vi "Select Pixel from MUX.vi"(7 "Cell position":dbl, 9 "Pixel":i32, 10 "Sample Holder":dbl) -> ()   [LabVIEW 2011]
uses:
  <vilib>/ULx/Create Channel.llb/ULx Create Channel (DO-Digital Output).vi
  <vilib>/ULx/Write.llb/ULx Write (Digital U32 1Chan 1Samp).vi
panel:
  in  "Port":refnum<k21>="Dev0/AuxPort"
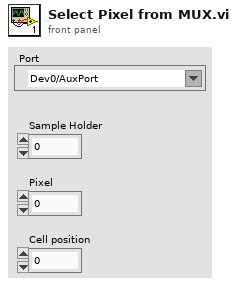
[diagram p1: front panel]
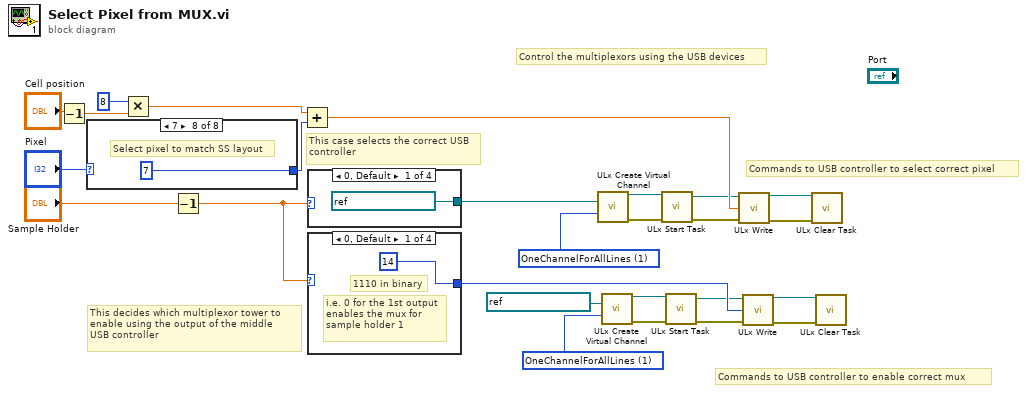
[diagram p0: block diagram]
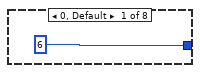
[diagram p2: hidden frame]
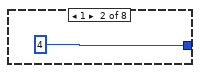
[diagram p3: hidden frame]
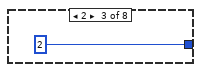
[diagram p4: hidden frame]
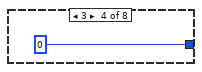
[diagram p5: hidden frame]
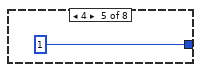
[diagram p6: hidden frame]
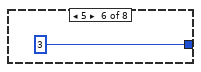
[diagram p7: hidden frame]
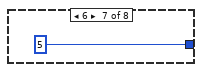
[diagram p8: hidden frame]
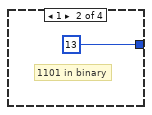
[diagram p9: hidden frame]
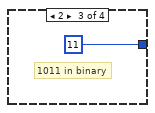
[diagram p10: hidden frame]
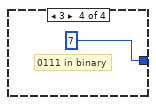
[diagram p11: hidden frame]
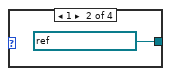
[diagram p12: hidden frame]
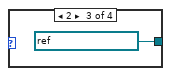
[diagram p13: hidden frame]
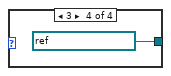
[diagram p14: hidden frame]
diagram:
  w15 = 1 items=["OneChannelForEachLine", "OneChannelForAllLines"] ("line grouping")
  w2 = 1 items=["OneChannelForEachLine", "OneChannelForAllLines"] ("line grouping")
  # "Control the multiplexors using the USB devices"
  # "Commands to USB controller to enable correct mux"
  # "Commands to USB controller to select correct pixel"
  # "This decides which multiplexor tower to\nenable using the output of the middle \nUSB controller"
  # "This case selects the correct USB\ncontroller"
  n1 = Decrement(x="Cell position") -> (x-1=w12:dbl)
  n2 = case shown="7" "Pixel" {
    tunnel: [6 4 2 0 1 3 5 7] -> w26
    frame 0, Default {
    }
    frame 1 {
    }
    frame 2 {
    }
    frame 3 {
    }
    frame 4 {
    }
    frame 5 {
    }
    frame 6 {
    }
    frame 7 {
      # "Select pixel to match SS layout"
    }
  }
  n3 = Multiply(x=8, y=w12) -> (x*y=w10:dbl)
  n4 = Decrement(x="Sample Holder") -> (x-1=w23:dbl)
  n5 = Add(x=w10, y=w26) -> (x+y=w13:dbl)
  n6 = case shown="0, Default" w23 {
    tunnel: [refnum<k21> "Dev0/1stPortA" ("Port 2") refnum<k21> "Dev0/1stPortB" ("Port 2") refnum<k21> "Dev1/1stPortA" ("Port 2") refnum<k21> "Dev1/1stPortB" ("Port 2")] -> w1
    frame 0, Default {
    }
    frame 1 {
    }
    frame 2 {
    }
    frame 3 {
    }
  }
  n7 = case shown="0, Default" w23 {
    tunnel: [14 13 11 7] -> w24
    frame 0, Default {
      # "i.e. 0 for the 1st output\nenables the mux for\nsample holder 1"
      # "1110 in binary"
    }
    frame 1 {
      # "1101 in binary"
    }
    frame 2 {
      # "1011 in binary"
    }
    frame 3 {
      # "0111 in binary"
    }
  }
  n8 = call-poly <vilib>:"ULx Create Virtual Channel.vi"("lines"=w1, "line grouping"=w2) -> ("task out"=w4:refnum<k24>, "error out"=w3:errorcluster)  [unwired: 12 in]
  n9 = call-poly <vilib>:"ULx Create Virtual Channel.vi"("lines"=refnum<k21> "Dev2/1stPortA" ("Port 2"), "line grouping"=w15) -> ("task out"=w17:refnum<k24>, "error out"=w16:errorcluster)  [unwired: 12 in]
  n10 = call <vilib>:"ULx Start Task.vi"("task in"=w4, "error in"=w3) -> ("task out"=w7:refnum<k24>, "error out"=w8:errorcluster)  [unwired: 12 in]
  n11 = call <vilib>:"ULx Start Task.vi"("task in"=w17, "error in"=w16) -> ("task out"=w20:refnum<k24>, "error out"=w21:errorcluster)  [unwired: 12 in]
  n12 = call-poly <vilib>:"ULx Write.vi"("task in"=w7, "data"=w13, "error in"=w8) -> ("task out"=w5:refnum<k24>, "error out"=w6:errorcluster)  [unwired: 10 in, 1 out]
  n13 = call-poly <vilib>:"ULx Write.vi"("task in"=w20, "data"=w24, "error in"=w21) -> ("task out"=w18:refnum<k24>, "error out"=w19:errorcluster)  [unwired: 10 in, 1 out]
  n14 = call <vilib>:"ULx Clear Task.vi"("task in"=w5, "error in"=w6) -> ()  [unwired: 13 in, 1 out]
  n15 = call <vilib>:"ULx Clear Task.vi"("task in"=w18, "error in"=w19) -> ()  [unwired: 13 in, 1 out]
